vi "Autoscale_Y_Multiple.vi"(11 "GraphRef":refnum<vi>) -> ()   [LabVIEW 2013]
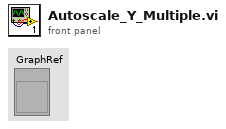
[diagram p1: front panel]
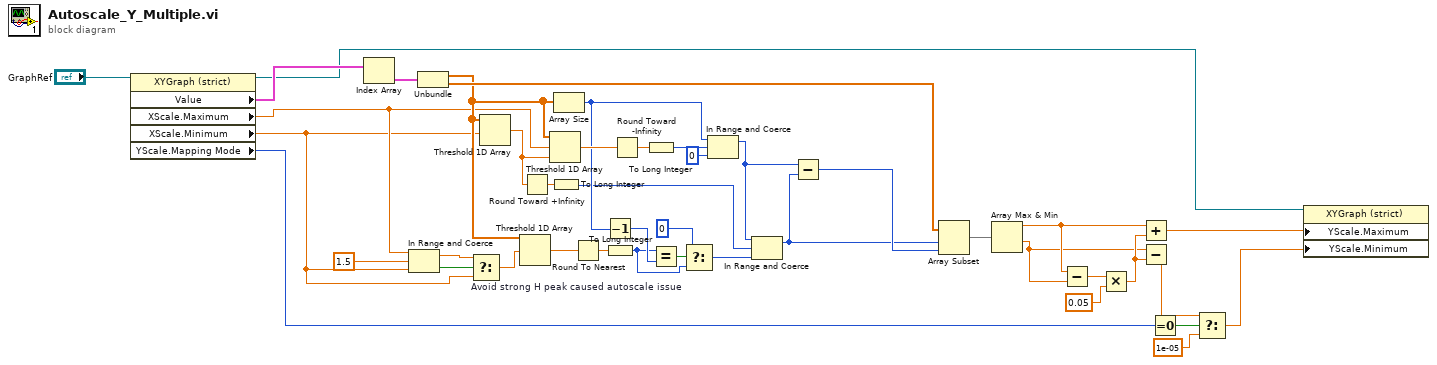
[diagram p0: block diagram]
diagram:
  n1 = property on="Property Node" class="XYGraph (strict)"(reference="GraphRef") -> (reference out=w14:refnum<vi>, "Value"=w42:cluster{dbl[], "Amplitudes":dbl[]}[], "XScale.Maximum"=w11:dbl, "XScale.Minimum"=w7:dbl, "YScale.Mapping Mode"=w1:u8)  [unwired: 1 in, 1 out]
  n2 = Index Array(array=w42) -> (element=w26:cluster{dbl[], "Amplitudes":dbl[]})  [unwired: 1 in]
  n3 = In Range and Coerce(upper limit=w11, x=1.5 ("threshold y"), lower limit=w7) -> (coerced(x)=w8:dbl, In Range?=w9:bool)
  n4 = Unbundle(w26) -> (w13:dbl[], "Amplitudes"=w25:dbl[])
  n5 = Select "Avoid strong H peak caused autoscale issue"(t=w8, s=w9, f=w7) -> (s? t:f=w6:dbl)
  n6 = Threshold 1D Array(2:w7, 3:w13) -> (0:w36:dbl)  [unwired: 1 in]
  n7 = Threshold 1D Array(2:w6, 3:w13) -> (0:w32:dbl)  [unwired: 1 in]
  n8 = Round Toward +Infinity(x=w36) -> (ceil(x): smallest int >= x=w34:dbl)
  n9 = Threshold 1D Array(1:w36, 2:w11, 3:w13) -> (0:w37:dbl)
  n10 = To Long Integer(number=w34) -> (32bit integer=w17:i32)
  n11 = Array Size(array=w13) -> (size(s)=w29:i32)
  n12 = Round To Nearest(number=w32) -> (nearest integer value=w30:dbl)
  n13 = Decrement(x=w29) -> (x-1=w28:i32)
  n14 = To Long Integer(number=w30) -> (32bit integer=w19:i32)
  n15 = Round Toward -Infinity(1:w37) -> (0:w23:dbl)
  n16 = To Long Integer(number=w23) -> (32bit integer=w21:i32)
  n17 = Equal?(x=w19, y=w28) -> (x = y?=w31:bool)
  n18 = Select(t=0, s=w31, f=w19) -> (s? t:f=w20:i32)
  n19 = In Range and Coerce(upper limit=w29, x=w21, lower limit=0) -> (coerced(x)=w18:i32)  [unwired: 1 out]
  n20 = In Range and Coerce(upper limit=w18, x=w17, lower limit=w20) -> (coerced(x)=w16:i32)  [unwired: 1 out]
  n21 = Subtract(x=w18, y=w16) -> (x-y=w35:i32)
  n22 = Array Subset(array=w25, index=w16, length=w35) -> (w33:dbl[])
  n23 = Array Max & Min(array=w33) -> (max value=w38:dbl, min value=w12:dbl)  [unwired: 2 out]
  n24 = Subtract(x=w38, y=w12) -> (x-y=w41:dbl)
  n25 = Multiply(x=w41, y=0.05) -> (x*y=w39:dbl)
  n26 = Add(x=w38, y=w39) -> (x+y=w24:dbl)
  n27 = Subtract(x=w12, y=w39) -> (x-y=w2:dbl)
  n28 = Equal To 0?(x=w1) -> (x = 0?=w5:bool)
  n29 = Select(t=w2, s=w5, f=1e-05) -> (s? t:f=w3:dbl)
  n30 = property on="Property Node" class="XYGraph (strict)"(reference=w14, "YScale.Maximum"=w24, "YScale.Minimum"=w3) -> ()  [unwired: 1 in, 2 out]
